vi "SetControllerEnqueuer.vi"(8 "error in (no error)":errorcluster, 10 "Controller Enqueuer":refnum<class "Message Enqueuer.lvclass">, 11 "Stage in":refnum<class "Stage.lvclass">) -> (0 "error out":errorcluster, 3 "Stage out":refnum<class "Stage.lvclass">)   [LabVIEW 2020, in "Stage.lvlib" / "Stage.lvclass"]
uses:
  Stage.lvclass
  <vilib>/ActorFramework/Message Enqueuer/Message Enqueuer.lvclass
  Stage.lvclass/Stage.ctl
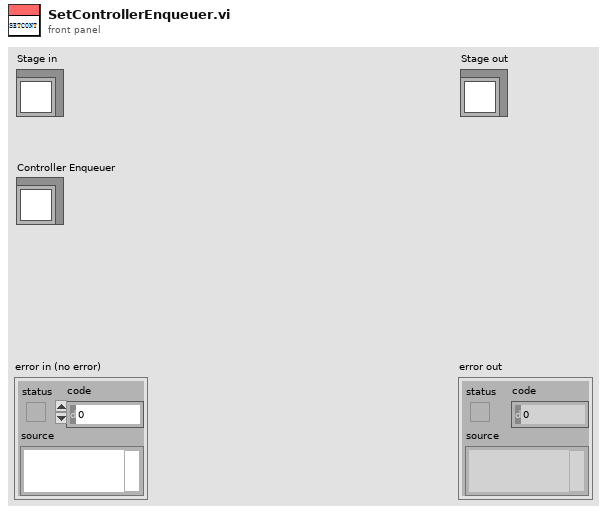
[diagram p1: front panel]
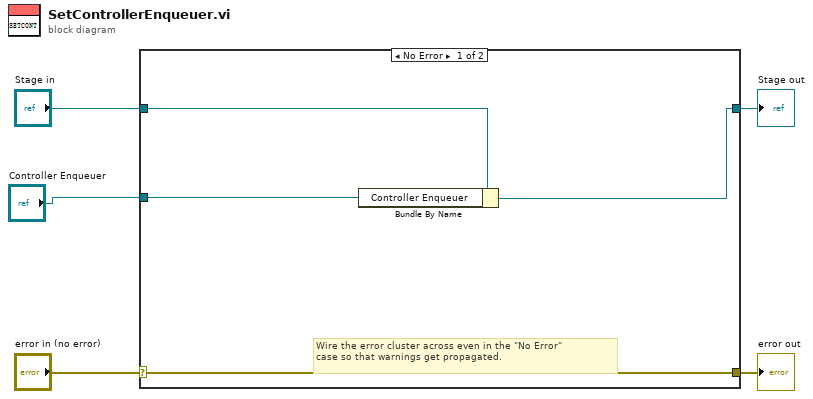
[diagram p0: block diagram]
diagram:
  n1 = case shown="No Error" "error in (no error)" {
    selector: "error in (no error)" -> [w9 w11]
    tunnel: [w9 w11] -> w4
    tunnel: [w7 w10] -> w2
    tunnel: "Stage in" -> [w8 w10]
    tunnel: "Controller Enqueuer" -> [w6 _]
    frame No Error {
      # "Wire the error cluster across even in the \"No Error\"\ncase so that warnings get propagated."
      n2 = Bundle By Name(cluster=w8, "Controller Enqueuer"=w6) -> (w7:refnum<class "Stage.lvclass">)
    }
    frame Error {
    }
  }
  "error out" <- w4
  "Stage out" <- w2
